vi "SENS_CORR_EXT_PORT_LOSS.vi"(0 "VISA IN":refnum<visa-resource-name>, 1 "Port":i32, 2 "Loss \"Use\" number":i32, 3 "Loss(dB)":i32, 5 "error in":errorcluster, 7 "Channel":i32) -> (14 "VISA Out":refnum<visa-resource-name>, 19 "error out":errorcluster)   [LabVIEW 2018, in "PNA-X.lvlib"]
doc: "SENSe<cnum>:CORRection:EXTension:PORT<pnum>:LOSS<n> <value> \n(Read-Write) Sets and returns the Loss value for the specified port number. \nLearn about Loss Compensation values. \nNote: This command affects ALL measurements on the specified channel. \nParameters \n<cnum> Any existing channel number. If unspecified, value is set to 1 \n<pnum> Port Number that will receive the Freq/Loss settings. If unspecified, value is set \nto 1. \n<n> Loss \"Use\" number. Choose from 1 or 2. If unspecified, value is set to 1. \n<value> Loss in dB. Choose a value between -90 and 90 \nExamples SENS:CORR:EXT:PORT:LOSS1 1 \nsense2:correction:extension:port2:loss2 .1 \nQuery Syntax SENSe<cnum>:CORRection:EXTension:PORT<pnum>:LOSS<n>? \nReturn Type Numeric \nDefault 0"
uses:
  PNA-X.lvlib
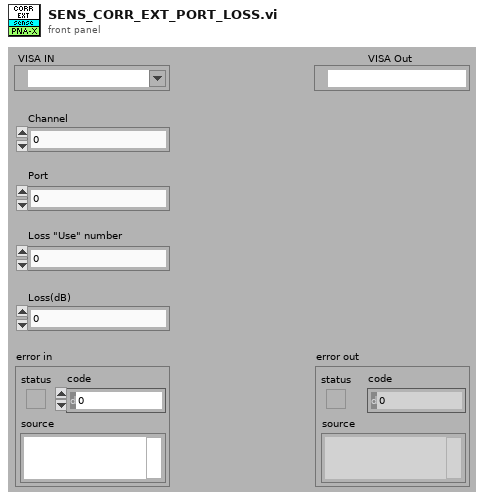
[diagram p1: front panel]
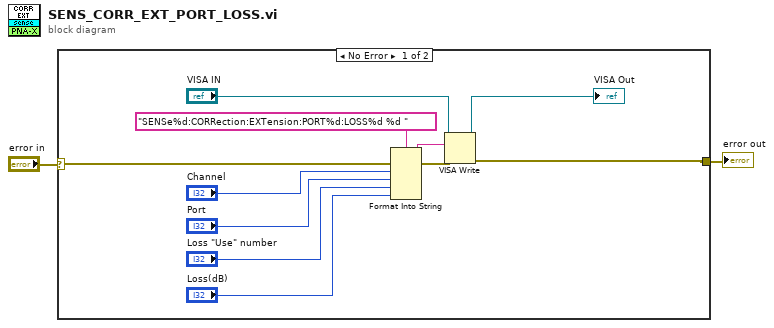
[diagram p0: block diagram]
diagram:
  n1 = case shown="No Error" "error in" {
    selector: "error in" -> [w13 w14]
    tunnel: [w8 w14] -> w1
    frame No Error {
      n2 = Format Into String(format string="SENSe%d:CORRection:EXTension:PORT%d:LOSS%d %d " ("Cmdline"), error in=w13, "Channel", "Port", "Loss \"Use\" number", "Loss(dB)") -> (resulting string=w11:string, error out=w12:errorcluster)  [unwired: 1 in]
      n3 = VISA Write(VISA resource name="VISA IN", write buffer=w11, error in (no error)=w12) -> (VISA resource name out=→"VISA Out":refnum<visa-resource-name>, error out=w8:errorcluster)  [unwired: 1 out]
    }
    frame Error {
    }
  }
  "error out" <- w1
